vi "WaitForGoodIPAddress.vi"() -> (0 "Good?":bool)   [LabVIEW 2012]
doc: "Wait for a valid IP address"
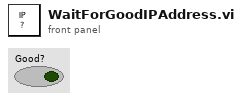
[diagram p1: front panel]
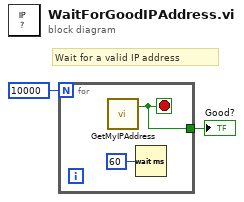
[diagram p0: block diagram]
diagram:
  # "Wait for a valid IP address"
  n1 = for {
    N: 10000 -> [_]
    tunnel: [w3] -> w2
    stop <- w3 stop-if-true
    n2 = call <userlib>:"GetMyIPAddress.vi"() -> ("Good?"=w3:bool)  [unwired: 2 in, 1 out]
    n3 = Wait (ms)(milliseconds to wait=u32 60) -> ()  [unwired: 1 out]
  }
  "Good?" <- w2
